vi "TEMPLATE.vi"(8 "error in (no error)":errorcluster, 11 "TestCase in":refnum<class "TestCurrentValueTable.lvclass">) -> (0 "error out":errorcluster, 3 "TestCase out":refnum<class "TestCurrentValueTable.lvclass">)   [LabVIEW 2015, in "CurrentValueTable.lvlib" / "TestCurrentValueTable.lvclass"]
uses:
  TestCurrentValueTable.lvclass
  <vilib>/addons/_JKI Toolkits/VI Tester/TestCase.llb/TestCase.lvclass
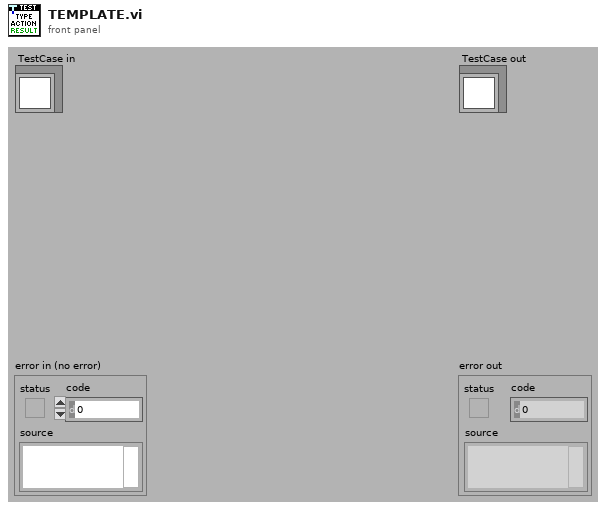
[diagram p1: front panel]
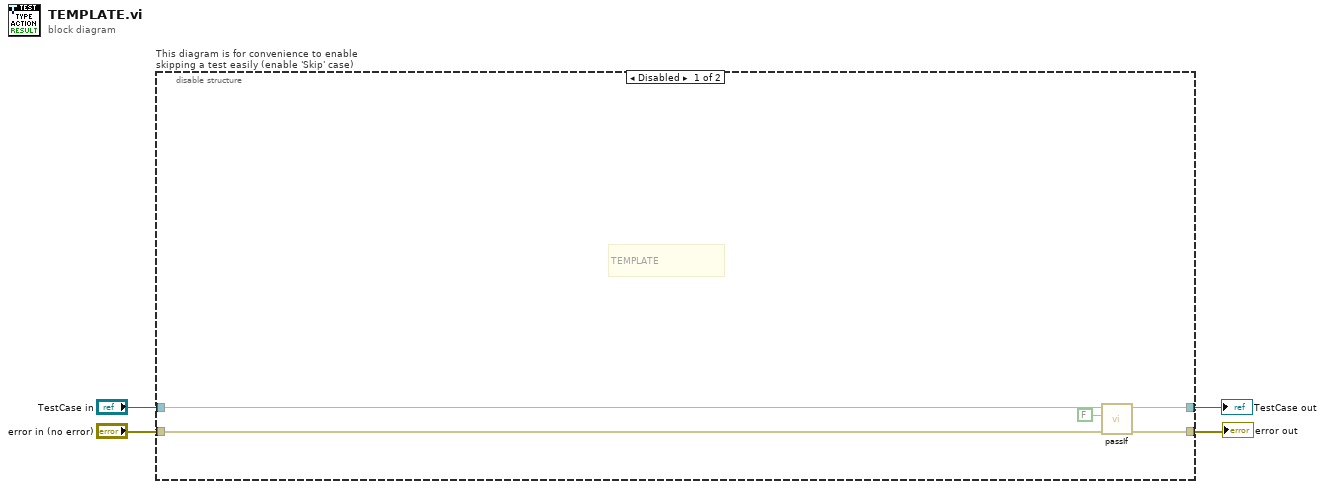
[diagram p0: block diagram]
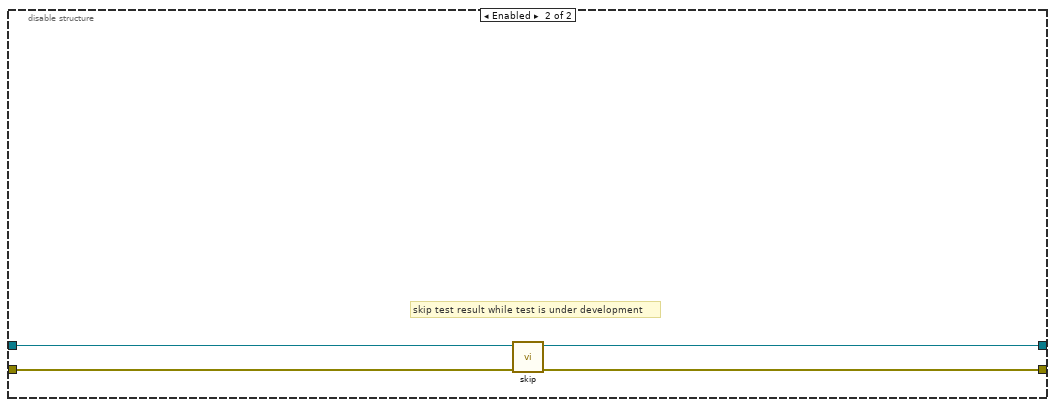
[diagram p2: hidden frame]
diagram:
  n1 = disable-structure "This diagram is for convenience to enable skipping a test easily (enable 'Skip' case)" shown="Disabled" {
    disable-tunnel: "TestCase in" -> [w9 w13]
    disable-tunnel: [w8 w11] -> w1
    disable-tunnel: [w7 w12] -> w3
    disable-tunnel: "error in (no error)" -> [w6 w10]
    frame Disabled {
      # "TEMPLATE"
      n2 = call-dynamic "passIf.vi"("error in (no error)"=w6, "pass"=FALSE, "TestCase in"=w9) -> ("error out"=w7:errorcluster, "TestCase out"=w8:refnum<class "TestCurrentValueTable.lvclass">)  [unwired: 7 in]
    }
    frame Enabled {
      # "skip test result while test is under development"
      n3 = call <vilib>:"skip.vi"("error in (no error)"=w10, "TestCase in"=w13) -> ("error out"=w12:errorcluster, "TestCase out"=w11:refnum<class "TestCurrentValueTable.lvclass">)  [unwired: 8 in]
    }
  }
  "error out" <- w3
  "TestCase out" <- w1
